vi "string match filter.vi"(10 "string filter value":string, 11 "channel value":string) -> (3 "Boolean":bool)   [LabVIEW 2016, in "FPGA Addon System Explorer.lvlib"]
uses:
  FPGA Addon System Explorer.lvlib
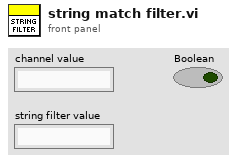
[diagram p1: front panel]
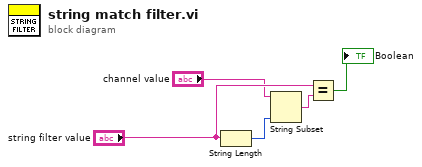
[diagram p0: block diagram]
diagram:
  n1 = String Length(string="string filter value") -> (length=w2:i32)
  n2 = String Subset(string="channel value", length (rest)=w2) -> (substring=w3:string)  [unwired: 1 in]
  n3 = Equal?(x="string filter value", y=w3) -> (x = y?=→"Boolean":bool)
